vi "handleSettings.vi"(8 "error in (no error)":errorcluster, 10 "Path":path, 11 "AndorController in":refnum<class "AndorController.lvclass">) -> (0 "error out":errorcluster, 3 "AndorController out":refnum<class "AndorController.lvclass">)   [LabVIEW 2009, in "Hardware.lvlib" / "Channels.lvlib" / "AndorController.lvclass"]
uses:
  AndorController.lvclass
  CameraEventsManager/CameraEventsManger.lvclass
  CameraAcquisitor.lvclass
  CameraSettingsViewer/andorSettingsViewer.lvclass
panel:
  in  "Tab Control":T1(tab)
  in  "acquisition_mode":u16(ring)=2 caption="Acquisition Mode" items=["Single Shot"=1, "Accumulative Series"=2, "Kinetic Series"=3, "Fast Kinetic Series"=4, "Run 'till Abort"=5]
  in  "readout_mode":i16(ring)=1 caption="Readout Mode" items=["Full Vertical Binning"=0, "Single Track"=3, "Multi-Track"=1, "Random Track"=2, "Full Resolusion Image"=4]
  in  "subArea_coordinate":i32(listbox) caption="SubArea Coordinates of top left corner"
  in  "vertical_binning":dbl=1.0 caption="Vertical Binning"
  in  "horizontal_binning":dbl=1.0 caption="Horizontal Binning"
  in  "subArea_height":dbl=1024.0 caption="SubArea Height"
  in  "subArea_width":dbl=1024.0 caption="SubArea Width"
  in  "offset":dbl caption="Offset"
  in  "number_tracks":i32 caption="Number of Tracks"
  in  "track_positions":i32(listbox) caption="Track Positions"
  in  "fast_kinetic_shift_speed":dbl caption="Fast Kinetic Shift Speed"
  in  "horizontal_shift_speed":enum16{"2.5", "1", "0.05"}(ring) caption="Horizontal Shift Speed"
  in  "vertical_shift_speed":T2(ring) caption="Vertical Shift Speed"
  in  "fast_kinetic_image_number":dbl=1.0 caption="Number in fast Kinetic Series"
  in  "fast_kinetic_cycle_time":dbl caption="Fast Kinetic Cycle Time"
  in  "accumulative_cycle_time":dbl caption="Accumulative Cycle Time"
  in  "kinetic_cycle_time":dbl caption="Kinetic Cycle Time"
  in  "accumulation_image_number":dbl=1.0 caption="Number of Accumulations"
  in  "kinetic_image_number":dbl=1.0 caption="Number in Kinetic Series"
  in  "mode":enum16{"Automatic", "Hold Open", "Hold Closed"}(ring) caption="Shutter Mode"
  in  "open_time":dbl=20.0 caption="Shutter Open Time"
  in  "close_time":dbl=20.0 caption="Shutter Close Time"
  in  "exposure_time":dbl=0.02 caption="Exposure Time"
  out "start_trigger":string caption="Trigger Channel"
  in  "trigger_mode":u16(ring) caption="Trigger Mode" items=["Internal"=0, "External"=1, "Fast External"=6]
  in  "fast_trigger":bool caption="Fast Triggering"
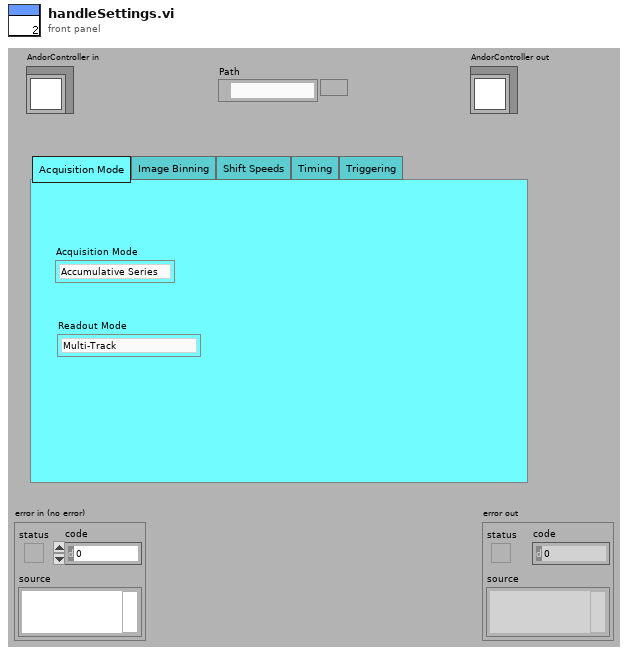
[diagram p1: front panel]
types:
  T1 = enum32{"modes", "image_binning", "shift_speeds", "timing", "triggering"}
  T2 = enum16{"0.525", "0.875", "1.575", "2.975", "5.775", "11.375", "22.575", "44.975"}
  T3 = cluster{"settingsFrontEndEvents":cluster{"loadSettingsFromPath":refnum<user-event>, "lookUpElementEvent":refnum<user-event>, "saveSettings":refnum<user-event>, "loadSettings":refnum<user-event>, "close":refnum<user-event>, "replaceElement":refnum<user-event>, "findParentNodes":refnum<user-event>, "createNode":refnum<user-event>}, "settingBackEndEvents":cluster{"defaultSettingsPathRequest":refnum<user-event>, "searchResultEvent":refnum<user-event>, "settingsSaved":refnum<user-event>, "settingsLoaded":refnum<user-event>, "foundParentNode":refnum<user-event>}}
  T4 = cluster{"loadSettingsFromPath":refnum<user-event>, "lookUpElementEvent":refnum<user-event>, "saveSettings":refnum<user-event>, "loadSettings":refnum<user-event>, "close":refnum<user-event>, "replaceElement":refnum<user-event>, "findParentNodes":refnum<user-event>, "createNode":refnum<user-event>}
  T5 = enum16{"Number", "String", "NumberArray", "StringArray", "xmlNode"}
  T6 = cluster{"[0]":dbl, "[1]":dbl, "[2]":dbl, "[3]":dbl}
  T7 = cluster{"[0]":dbl, "[1]":dbl, "[2]":dbl, "[3]":dbl, "[0]":dbl, "[1]":dbl, cluster{"[0]":i32, "[1]":i32}[], i32[]}
  T8 = cluster{"[0]":dbl, "[1]":dbl, "[2]":dbl, "[3]":dbl, "[4]":dbl, "[5]":dbl, "[6]":dbl}
  T9 = cluster{"[0]":dbl, "[1]":dbl, "[2]":dbl, "[3]":dbl, "[4]":dbl, "[5]":dbl, "[6]":dbl, dbl}
  T10 = cluster{"shutter Open Time":dbl, "Shutter Close Time":dbl, "Exposure Time":dbl, " AccumulatedCycleTime":dbl, " KineticCycleTime":dbl, "Number of Accumulations":dbl, "Number in Kinetic Series ":dbl, "Shutter Mode":dbl}
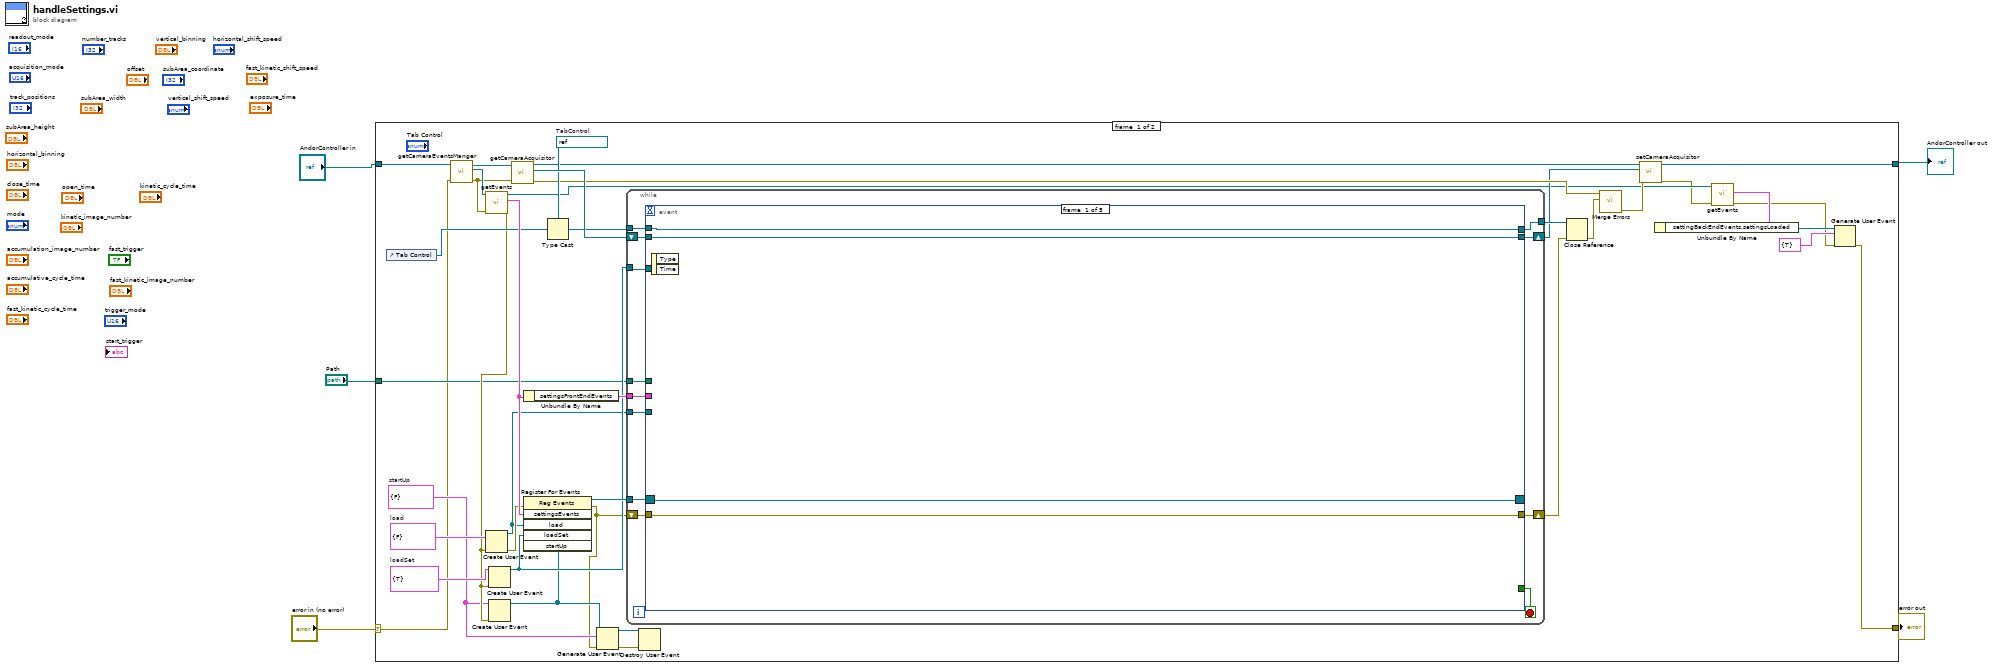
[diagram p0: block diagram]
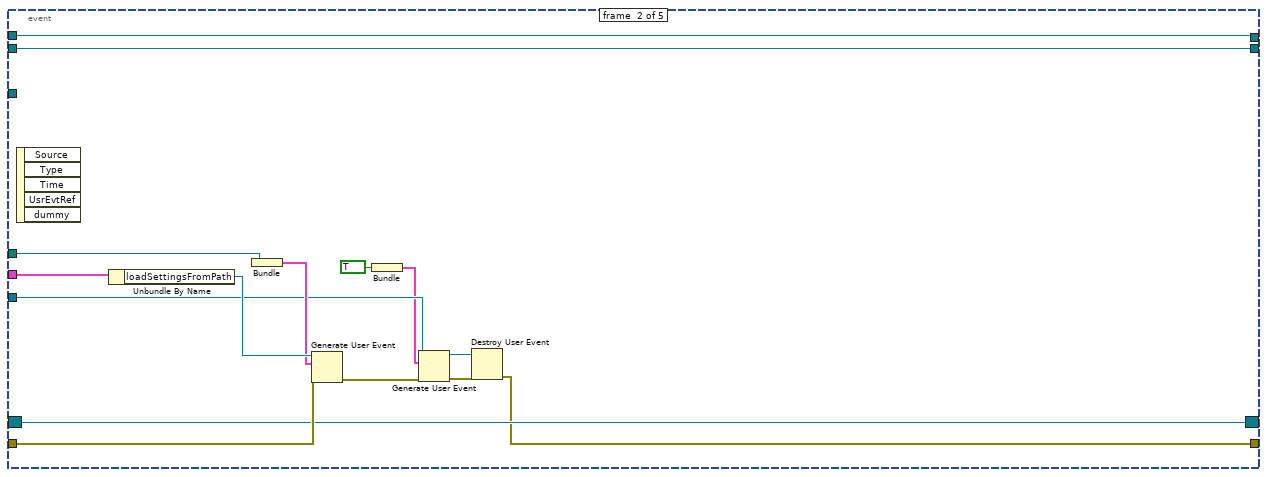
[diagram p2: hidden frame]
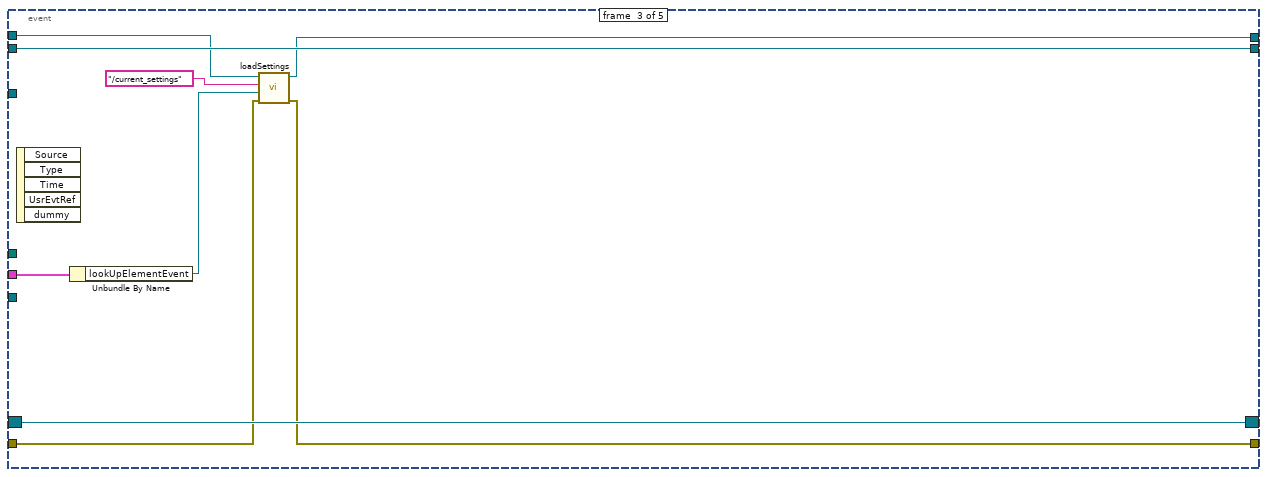
[diagram p3: hidden frame]
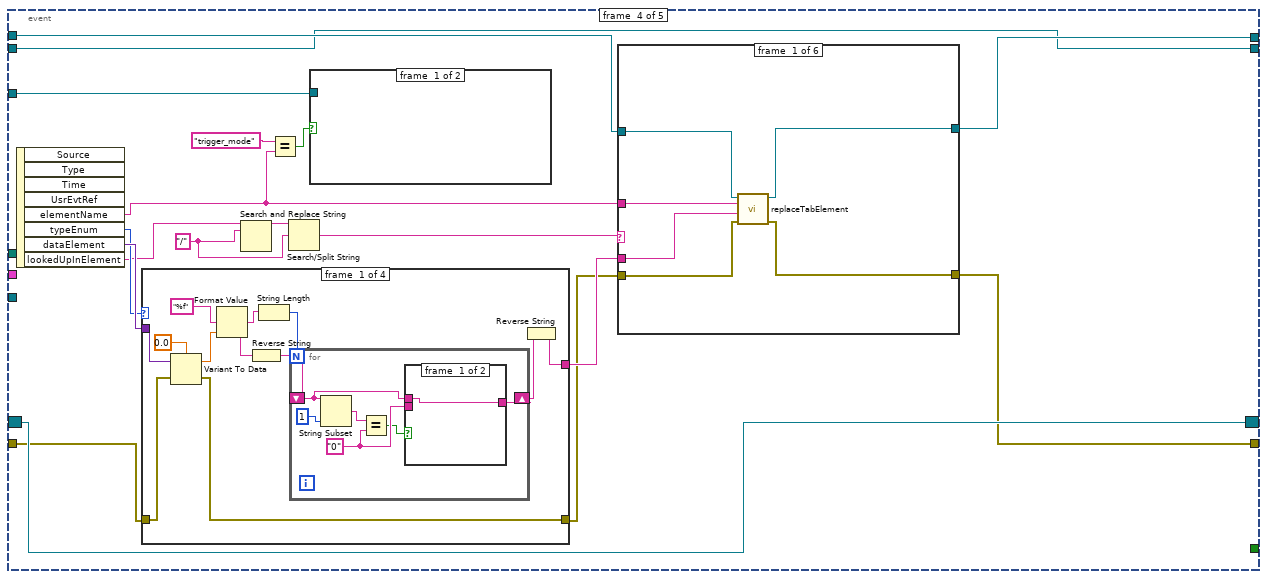
[diagram p4: hidden frame]
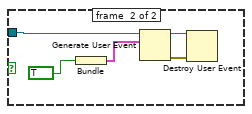
[diagram p5: hidden frame]
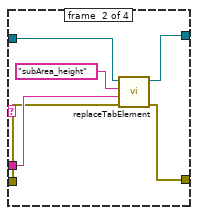
[diagram p7: hidden frame]
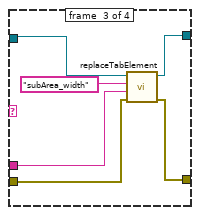
[diagram p8: hidden frame]
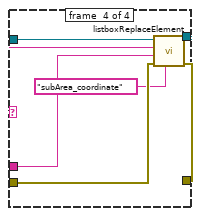
[diagram p9: hidden frame]
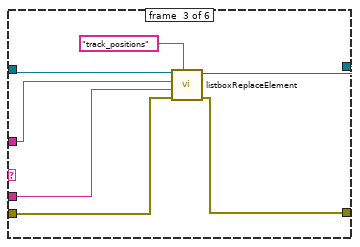
[diagram p10: hidden frame]
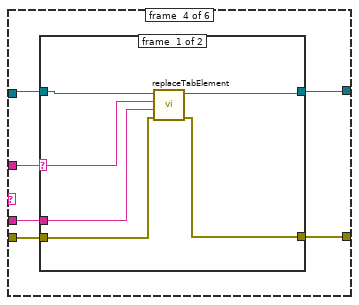
[diagram p11: hidden frame]
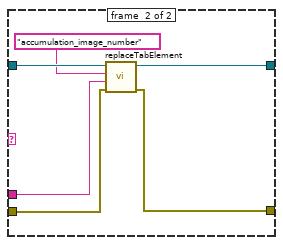
[diagram p12: hidden frame]
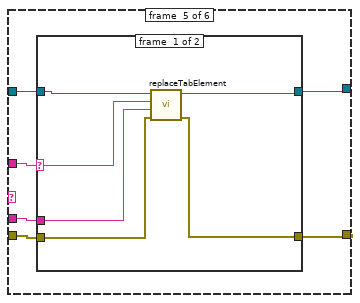
[diagram p13: hidden frame]
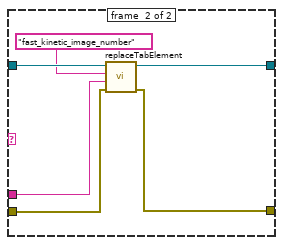
[diagram p14: hidden frame]
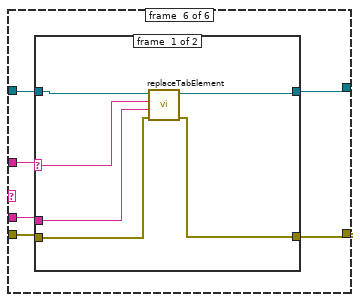
[diagram p15: hidden frame]
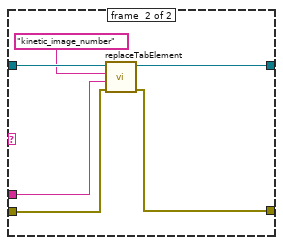
[diagram p16: hidden frame]
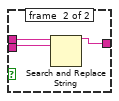
[diagram p17: hidden frame]
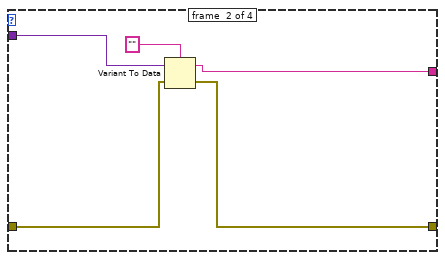
[diagram p18: hidden frame]
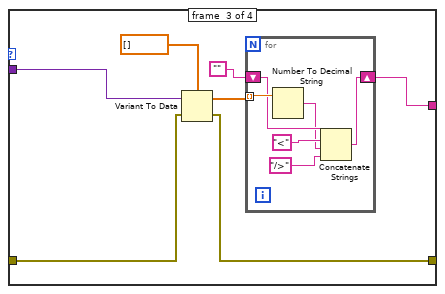
[diagram p19: hidden frame]
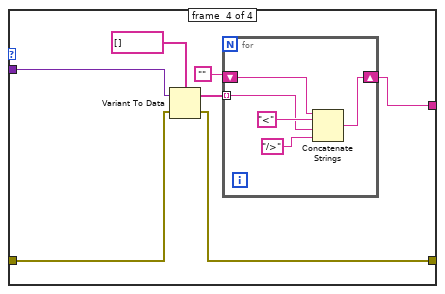
[diagram p20: hidden frame]
diagram:
  n1 = case shown="No Error" "error in (no error)" {
    selector: "error in (no error)" -> [w13 w478]
    tunnel: [w6 w478] -> w2
    tunnel: [w15 w477] -> w1
    tunnel: "AndorController in" -> [w14 w477]
    tunnel: "Path" -> [w23 _]
    frame #0 {
      w27 = cluster{"dummy":bool} {"dummy"=FALSE}  # startUp
      w33 = cluster{"dummy":bool} {"dummy"=TRUE}  # loadSet
      w36 = refnum<vi> refnum  # TabControl
      w37 = cluster{"dummy":bool} {"dummy"=FALSE}  # load
      n2 = control-ref of="Tab Control"() -> (w35:refnum<vi>)
      n3 = call-dynamic "getCameraEventsManger.vi"("error in (no error)"=w13, "CameraController.lvclass in"=w14) -> ("error out"=w39:errorcluster, "Hardware:Channels.lvlib:CameraEventsManger.lvclass"=w44:refnum<class "CameraEventsManger.lvclass">, "CameraController.lvclass out"=w40:refnum<class "AndorController.lvclass">)  [unwired: 7 in]
      n4 = call-dynamic "getEvents.vi"("error in (no error)"=w39, "CameraEventsManger in"=w44) -> ("error out"=w30:errorcluster, "settingsEvents"=w42:T3, "CameraEventsManger out"=w12:refnum<class "CameraEventsManger.lvclass">)  [unwired: 5 in, 2 out]
      n5 = Create User Event(user event datatype=w37, error in=w30) -> (user event=w29:refnum<user-event>, error out=w32:errorcluster)
      n6 = Create User Event(user event datatype=w33, error in=w30) -> (user event=w31:refnum<user-event>)  [unwired: 1 out]
      n7 = Create User Event(user event datatype=w27, error in=w30) -> (user event=w28:refnum<user-event>)  [unwired: 1 out]
      n8 = call-dynamic "getCameraAcquisitor.vi"("error in (no error)"=w39, "CameraController.lvclass in"=w40) -> ("error out"=w20:errorcluster, "CameraAcquisitor.lvclass"=w38:refnum<class "CameraAcquisitor.lvclass">, "CameraController.lvclass out"=w21:refnum<class "AndorController.lvclass">)  [unwired: 7 in]
      n9 = Unbundle By Name(w42) -> ("settingsFrontEndEvents"=w41:T4)
      n10 = register-events(error in=w32, w42, w29, w31, w28) -> (reference out=w43:refnum<event-registration>, error out=w26:errorcluster)  [unwired: 1 in]
      n11 = Type Cast(type=w36, x=w35) -> (*(type *) &x=w34:refnum<vi>)
      n12 = Generate User Event(user event=w28, event data cluster=w27, error in=w26) -> (user event out=w24:refnum<user-event>, error out=w25:errorcluster)
      n13 = while {
        tunnel: w43 -> [w56]
        shift-right: [w53] -> w18
        shift-left: w26 -> [w55]
        tunnel: w41 -> [w54]
        shift-right: [w51] -> w17
        shift-left: w38 -> [w52]
        tunnel: w29 -> [w50]
        tunnel: w34 -> [w49]
        tunnel: [w48] -> w22
        tunnel: w31 -> [w46]
        tunnel: w23 -> [w45]
        stop <- w47 stop-if-true
        n14 = event shown="[4] <loadSet>: User Event" {
          selector: w56 -> [w59 w71 w84 w102 w253]
          dyn-events: [w59 w71 w84 w102 w253] -> _
          timeout: _ -> [_ _ _ _ _]
          tunnel: w55 -> [w58 w72 w78 w100 w260]
          tunnel: w54 -> [_ w75 w80 _ _]
          tunnel: [w58 w62 w77 w93 w255] -> w53
          tunnel: w52 -> [w60 w70 w83 w94 w259]
          tunnel: [w60 w70 w83 w94 w257] -> w51
          tunnel: w50 -> [_ w69 _ _ _]
          tunnel: w49 -> [w57 w65 w82 w98 w261]
          tunnel: [w57 w65 w76 w95 w258] -> w48
          tunnel: [_ _ _ _ TRUE] -> w47
          tunnel: w46 -> [_ _ _ w89 _]
          tunnel: w45 -> [_ w64 _ _ _]
          event #0 {
            n15 = event-data() -> ()  [unwired: 1 in, 2 out]
          }
          event #1 {
            n16 = event-data() -> ()  [unwired: 1 in, 5 out]
            n17 = Unbundle By Name(w75) -> ("loadSettingsFromPath"=w74:refnum<user-event>)
            n18 = Bundle("Path"=w64) -> (w73:cluster{"Path":path})  [unwired: 1 in]
            n19 = Generate User Event(user event=w74, event data cluster=w73, error in=w72) -> (error out=w66:errorcluster)  [unwired: 1 out]
            n20 = Bundle(TRUE) -> (w67:cluster{bool})  [unwired: 1 in]
            n21 = Generate User Event(user event=w69, event data cluster=w67, error in=w66) -> (user event out=w61:refnum<user-event>, error out=w63:errorcluster)
            n22 = Destroy User Event(user event=w61, error in=w63) -> (error out=w62:errorcluster)
          }
          event #2 {
            n23 = event-data() -> ()  [unwired: 1 in, 5 out]
            n24 = Unbundle By Name(w80) -> ("lookUpElementEvent"=w79:refnum<user-event>)
            n25 = call "loadSettings.vi"("error in (no error)"=w78, "lookUpElementEvent"=w79, "whichSettings"="/current_settings", "TabCtl Refnum in"=w82) -> ("error out"=w77:errorcluster, "TabCtl Refnum out"=w76:refnum<vi>)  [unwired: 6 in]
          }
          event #3 {
            w87 = "/"
            n26 = event-data() -> ("elementName"=w91:string, "typeEnum"=w99:T5, "dataElement"=w101:variant, "lookedUpInElement"=w86:string)  [unwired: 1 in, 4 out]
            n27 = case shown="\"Number\", Default" w99 {
              tunnel: w101 -> [w209 w227 w233 w247]
              tunnel: w100 -> [w210 w226 w232 w246]
              tunnel: [w211 w225 w231 w241] -> w96
              tunnel: [w203 w223 w228 w242] -> w97
              frame #0 {
                n28 = Variant To Data(error in=w210, Variant=w209, type=0.0) -> (error out=w211:errorcluster, data=w202:dbl)
                n29 = Format Value(format string="%f", value (0)=w202) -> (output string=w205:string)  [unwired: 1 in]
                n30 = Reverse String(1:w205) -> (0:w207:string)
                n31 = String Length(string=w205) -> (length=w206:i32)
                n32 = for {
                  N: w206 -> [_]
                  shift-right: [w213] -> w204
                  shift-left: w207 -> [w216]
                  w215 = "0"
                  n33 = String Subset(string=w216, length (rest)=1) -> (substring=w217:string)  [unwired: 1 in]
                  n34 = Equal?(x=w217, y=w215) -> (x = y?=w214:bool)
                  n35 = case shown="True" w214 {
                    tunnel: w216 -> [w219 w222]
                    tunnel: w215 -> [_ w220]
                    tunnel: [w219 w221] -> w213
                    frame #0 {
                    }
                    frame #1 {
                      n36 = Search and Replace String(input string=w222, search string=w220) -> (result string=w221:string)  [unwired: 6 in, 3 out]
                    }
                  }
                }
                n37 = Reverse String(1:w204) -> (0:w203:string)
              }
              frame #1 {
                n38 = Variant To Data(error in=w226, Variant=w227, type="") -> (error out=w225:errorcluster, data=w223:string)
              }
              frame #2 {
                n39 = Variant To Data(error in=w232, Variant=w233, type=dbl[] []) -> (error out=w231:errorcluster, data=w230:dbl[])
                n40 = for {
                  tunnel: w230 -> [w240] mode=indexing
                  shift-right: [w235] -> w228
                  shift-left: "" -> [w239]
                  n41 = Number To Decimal String(number=w240) -> (decimal integer string=w237:string)  [unwired: 1 in]
                  n42 = Concatenate Strings(w239, "<", w237, "/>") -> (w235:string)
                }
              }
              frame #3 {
                n43 = Variant To Data(error in=w246, Variant=w247, type=string[] []) -> (error out=w241:errorcluster, data=w244:string[])
                n44 = for {
                  shift-right: [w248] -> w242
                  shift-left: "" -> [w249]
                  tunnel: w244 -> [w250] mode=indexing
                  n45 = Concatenate Strings(w249, "<", w250, "/>") -> (w248:string)
                }
              }
            }
            n46 = Search and Replace String(input string=w86, search string=w87) -> (result string=w88:string)  [unwired: 6 in, 3 out]
            n47 = Equal?(x="trigger_mode", y=w91) -> (x = y?=w90:bool)
            n48 = Search/Split String(string=w88, search string/char (-)=w87) -> (match + rest of string=w85:string)  [unwired: 1 in, 2 out]
            n49 = case shown="True" w90 {
              tunnel: w89 -> [_ w107]
              frame #0 {
              }
              frame #1 {
                n50 = Bundle(TRUE) -> (w105:cluster{bool})  [unwired: 1 in]
                n51 = Generate User Event(user event=w107, event data cluster=w105) -> (user event out=w103:refnum<user-event>, error out=w104:errorcluster)  [unwired: 1 in]
                n52 = Destroy User Event(user event=w103, error in=w104) -> ()  [unwired: 1 out]
              }
            }
            n53 = case shown="\"False\", Default" w85 {
              tunnel: w91 -> [w112 w114 w145 w151 w169 w187]
              tunnel: w98 -> [w113 w115 w147 w153 w171 w189]
              tunnel: w97 -> [w111 w119 w144 w152 w170 w188]
              tunnel: w96 -> [w110 w118 w142 w148 w166 w184]
              tunnel: [w109 w117 w141 w149 w167 w185] -> w93
              tunnel: [w108 w116 w146 w150 w168 w186] -> w95
              frame #0 {
                n54 = call "replaceTabElement.vi"("error in (no error)"=w110, "replaceWith"=w111, "replaceElementLabeled"=w112, "Tab ref in"=w113) -> ("error out"=w109:errorcluster, "Tab ref out"=w108:refnum<vi>)  [unwired: 6 in]
              }
              frame #1 {
                n55 = case shown="\"width\"" w114 {
                  selector: w114 -> [_ _ _ w135]
                  tunnel: w119 -> [_ w127 w129 w136]
                  tunnel: w118 -> [w120 w126 w130 w138]
                  tunnel: [w120 w125 w131 w137] -> w117
                  tunnel: [w121 w124 w132 w139] -> w116
                  tunnel: w115 -> [w121 w123 w133 w140]
                  frame #0 {
                  }
                  frame #1 {
                    n56 = call "replaceTabElement.vi"("error in (no error)"=w126, "replaceWith"=w127, "replaceElementLabeled"="subArea_height", "Tab ref in"=w123) -> ("error out"=w125:errorcluster, "Tab ref out"=w124:refnum<vi>)  [unwired: 6 in]
                  }
                  frame #2 {
                    n57 = call "replaceTabElement.vi"("error in (no error)"=w130, "replaceWith"=w129, "replaceElementLabeled"="subArea_width", "Tab ref in"=w133) -> ("error out"=w131:errorcluster, "Tab ref out"=w132:refnum<vi>)  [unwired: 6 in]
                  }
                  frame #3 {
                    n58 = call "listboxReplaceElement.vi"("inElement"="subArea_coordinate", "error in (no error)"=w138, "replaceElementWith"=w136, "elementName"=w135, "TabCtl Refnum"=w140) -> ("error out"=w137:errorcluster, "TabCtl Refnum out"=w139:refnum<vi>)  [unwired: 5 in]
                  }
                }
              }
              frame #2 {
                n59 = call "listboxReplaceElement.vi"("inElement"="track_positions", "error in (no error)"=w142, "replaceElementWith"=w144, "elementName"=w145, "TabCtl Refnum"=w147) -> ("error out"=w141:errorcluster, "TabCtl Refnum out"=w146:refnum<vi>)  [unwired: 5 in]
              }
              frame #3 {
                n60 = case shown="\"image_number\"" w151 {
                  selector: w151 -> [w158 _]
                  tunnel: w153 -> [w159 w165]
                  tunnel: w152 -> [w157 w164]
                  tunnel: [w154 w162] -> w150
                  tunnel: [w155 w161] -> w149
                  tunnel: w148 -> [w156 w160]
                  frame #0 {
                    n61 = call "replaceTabElement.vi"("error in (no error)"=w156, "replaceWith"=w157, "replaceElementLabeled"=w158, "Tab ref in"=w159) -> ("error out"=w155:errorcluster, "Tab ref out"=w154:refnum<vi>)  [unwired: 6 in]
                  }
                  frame #1 {
                    n62 = call "replaceTabElement.vi"("error in (no error)"=w160, "replaceWith"=w164, "replaceElementLabeled"="accumulation_image_number", "Tab ref in"=w165) -> ("error out"=w161:errorcluster, "Tab ref out"=w162:refnum<vi>)  [unwired: 6 in]
                  }
                }
              }
              frame #4 {
                n63 = case shown="\"image_number\"" w169 {
                  selector: w169 -> [w176 _]
                  tunnel: w171 -> [w177 w183]
                  tunnel: w170 -> [w175 w182]
                  tunnel: [w172 w180] -> w168
                  tunnel: [w173 w179] -> w167
                  tunnel: w166 -> [w174 w178]
                  frame #0 {
                    n64 = call "replaceTabElement.vi"("error in (no error)"=w174, "replaceWith"=w175, "replaceElementLabeled"=w176, "Tab ref in"=w177) -> ("error out"=w173:errorcluster, "Tab ref out"=w172:refnum<vi>)  [unwired: 6 in]
                  }
                  frame #1 {
                    n65 = call "replaceTabElement.vi"("error in (no error)"=w178, "replaceWith"=w182, "replaceElementLabeled"="fast_kinetic_image_number", "Tab ref in"=w183) -> ("error out"=w179:errorcluster, "Tab ref out"=w180:refnum<vi>)  [unwired: 6 in]
                  }
                }
              }
              frame #5 {
                n66 = case shown="\"False\", Default" w187 {
                  selector: w187 -> [w194 _]
                  tunnel: w189 -> [w195 w201]
                  tunnel: w188 -> [w193 w200]
                  tunnel: [w190 w198] -> w186
                  tunnel: [w191 w197] -> w185
                  tunnel: w184 -> [w192 w196]
                  frame #0 {
                    n67 = call "replaceTabElement.vi"("error in (no error)"=w192, "replaceWith"=w193, "replaceElementLabeled"=w194, "Tab ref in"=w195) -> ("error out"=w191:errorcluster, "Tab ref out"=w190:refnum<vi>)  [unwired: 6 in]
                  }
                  frame #1 {
                    n68 = call "replaceTabElement.vi"("error in (no error)"=w196, "replaceWith"=w200, "replaceElementLabeled"="kinetic_image_number", "Tab ref in"=w201) -> ("error out"=w197:errorcluster, "Tab ref out"=w198:refnum<vi>)  [unwired: 6 in]
                  }
                }
              }
            }
          }
          event #4 {
            n69 = event-data() -> ()  [unwired: 1 in, 5 out]
            n70 = for {
              N: 3 -> [_]
              shift-right: [w263] -> w258
              shift-left: w261 -> [w267]
              shift-right: [w262] -> w255
              shift-left: w260 -> [w266]
              shift-right: [w264] -> w257
              shift-left: w259 -> [w265]
              i -> [w268]
              n71 = case shown="1" w268 {
                tunnel: w267 -> [w269 w346 w398 w473]
                tunnel: w266 -> [w270 w345 w397 w443]
                tunnel: w265 -> [w271 w331 w370 w457]
                tunnel: [w271 w283 w369 w429] -> w264
                tunnel: [w269 w282 w375 w440] -> w263
                tunnel: [w270 w280 w371 w428] -> w262
                frame #0 {
                }
                frame #1 {
                  w297 = refnum<vi> refnum  # MulticolumnListbox
                  w302 = refnum<vi> refnum  # MulticolumnListbox
                  n72 = call "findTabElement.vi"("error in (no error)"=w345, "replaceElementLabeled"="acquisition_mode", "Tab ref in"=w346) -> ("error out"=w341:errorcluster, "Tab Control"=w337:refnum<vi>, "Tab ref out"=w343:refnum<vi>)  [unwired: 5 in, 1 out]
                  n73 = call "findTabElement.vi"("error in (no error)"=w341, "replaceElementLabeled"="readout_mode", "Tab ref in"=w343) -> ("error out"=w339:errorcluster, "Tab Control"=w336:refnum<vi>, "Tab ref out"=w340:refnum<vi>)  [unwired: 5 in, 1 out]
                  n74 = Build Array(w337, w336) -> (w332:refnum<vi>[])
                  n75 = call "findTabElement.vi"("error in (no error)"=w339, "replaceElementLabeled"="vertical_binning", "Tab ref in"=w340) -> ("error out"=w334:errorcluster, "Tab Control"=w312:refnum<vi>, "Tab ref out"=w335:refnum<vi>)  [unwired: 5 in, 1 out]
                  n76 = for {
                    tunnel: w332 -> [w357] mode=indexing
                    tunnel: [w356] -> w278 mode=indexing
                    n77 = call "getNumber.vi"("Tab Control"=w357) -> ("Number"=w356:dbl)  [unwired: 9 in, 1 out]
                  }
                  n78 = call "findTabElement.vi"("error in (no error)"=w334, "replaceElementLabeled"="horizontal_binning", "Tab ref in"=w335) -> ("error out"=w330:errorcluster, "Tab Control"=w311:refnum<vi>, "Tab ref out"=w328:refnum<vi>)  [unwired: 5 in, 1 out]
                  n79 = call "findTabElement.vi"("error in (no error)"=w330, "replaceElementLabeled"="subArea_height", "Tab ref in"=w328) -> ("error out"=w326:errorcluster, "Tab Control"=w310:refnum<vi>, "Tab ref out"=w327:refnum<vi>)  [unwired: 5 in, 1 out]
                  n80 = Index Array(array=w278) -> (element=w277:dbl)  [unwired: 1 in]
                  n81 = Index Array(array=w278, index=1) -> (element=w276:dbl)
                  n82 = call "findTabElement.vi"("error in (no error)"=w326, "replaceElementLabeled"="subArea_width", "Tab ref in"=w327) -> ("error out"=w324:errorcluster, "Tab Control"=w309:refnum<vi>, "Tab ref out"=w322:refnum<vi>)  [unwired: 5 in, 1 out]
                  n83 = Build Array(w312, w311, w310, w309) -> (w307:refnum<vi>[])
                  n84 = Bundle("Number"=w277, "Number"=w276, 0.0) -> (w274:cluster{"Number":dbl, "Number":dbl, dbl})  [unwired: 1 in]
                  n85 = call "findTabElement.vi"("error in (no error)"=w324, "replaceElementLabeled"="subArea_coordinate", "Tab ref in"=w322) -> ("error out"=w320:errorcluster, "Tab Control"=w303:refnum<vi>, "Tab ref out"=w321:refnum<vi>)  [unwired: 5 in, 1 out]
                  n86 = Type Cast(type=w302, x=w303) -> (*(type *) &x=w304:refnum<vi>)
                  n87 = for {
                    tunnel: w307 -> [w355] mode=indexing
                    tunnel: [w354] -> w308 mode=indexing
                    n88 = call "getNumber.vi"("Tab Control"=w355) -> ("Number"=w354:dbl)  [unwired: 9 in, 1 out]
                  }
                  n89 = call "findTabElement.vi"("error in (no error)"=w320, "replaceElementLabeled"="offset", "Tab ref in"=w321) -> ("error out"=w316:errorcluster, "Tab Control"=w273:refnum<vi>, "Tab ref out"=w317:refnum<vi>)  [unwired: 5 in, 1 out]
                  n90 = property class="MCListbox"(reference=w304) -> ("ItemNames"=w301:string[][])  [unwired: 1 in, 2 out]
                  n91 = call "findTabElement.vi"("error in (no error)"=w316, "replaceElementLabeled"="number_tracks", "Tab ref in"=w317) -> ("error out"=w314:errorcluster, "Tab Control"=w272:refnum<vi>, "Tab ref out"=w315:refnum<vi>)  [unwired: 5 in, 1 out]
                  n92 = Array To Cluster(array=w308) -> (cluster=w294:T6)
                  n93 = Build Array(w273, w272) -> (w305:refnum<vi>[])
                  n94 = call "findTabElement.vi"("error in (no error)"=w314, "replaceElementLabeled"="track_positions", "Tab ref in"=w315) -> ("error out"=w281:errorcluster, "Tab Control"=w295:refnum<vi>, "Tab ref out"=w282:refnum<vi>)  [unwired: 5 in, 1 out]
                  n95 = Type Cast(type=w297, x=w295) -> (*(type *) &x=w298:refnum<vi>)
                  n96 = Decimal String To Number(string=w301) -> (number=w300:i32[][])  [unwired: 2 in, 1 out]
                  n97 = property class="MCListbox"(reference=w298) -> ("ItemNames"=w296:string[][])  [unwired: 1 in, 2 out]
                  n98 = for {
                    tunnel: w305 -> [w353] mode=indexing
                    tunnel: [w352] -> w306 mode=indexing
                    n99 = call "getNumber.vi"("Tab Control"=w353) -> ("Number"=w352:dbl)  [unwired: 9 in, 1 out]
                  }
                  n100 = Reshape Array(w300, 2) -> (w285:i32[])
                  n101 = Array To Cluster(array=w306) -> (cluster=w293:cluster{"[0]":dbl, "[1]":dbl})
                  n102 = for {
                    tunnel: w296 -> [w351] mode=indexing
                    tunnel: [w347] -> w286 mode=indexing
                    n103 = Decimal String To Number(string=w351) -> (number=w350:i32[])  [unwired: 2 in, 1 out]
                    n104 = Reshape Array(w350, 2) -> (w348:i32[])
                    n105 = Array To Cluster(array=w348) -> (cluster=w347:cluster{"[0]":i32, "[1]":i32})
                  }
                  n106 = Unbundle(w293) -> ("[0]"=w288:dbl, "[1]"=w287:dbl)
                  n107 = Unbundle(w294) -> ("[0]"=w292:dbl, "[1]"=w291:dbl, "[2]"=w290:dbl, "[3]"=w289:dbl)
                  n108 = Bundle("[0]"=w292, "[1]"=w291, "[2]"=w290, "[3]"=w289, "[0]"=w288, "[1]"=w287, w286, w285) -> (w284:T7)  [unwired: 1 in]
                  n109 = call "configureImageAcquisition.vi"("error in (no error)"=w281, "Image Binning"=w284, "Mode"=w274, "CameraAcquisitor in"=w331) -> ("error out"=w280:errorcluster, "CameraAcquisitor out"=w283:refnum<class "CameraAcquisitor.lvclass">)  [unwired: 6 in]
                }
                frame #2 {
                  w390 = refnum<vi> refnum  # Enum
                  n110 = Build Array("open_time", "close_time", "exposure_time", "accumulative_cycle_time", "kinetic_cycle_time", "accumulation_image_number", "kinetic_image_number") -> (w399:string[])
                  n111 = for {
                    tunnel: w399 -> [w424] mode=indexing
                    shift-right: [w418] -> w395
                    shift-left: w398 -> [w425]
                    shift-right: [w419] -> w393
                    shift-left: w397 -> [w423]
                    tunnel: [w420] -> w396 mode=indexing
                    n112 = call "findTabElement.vi"("error in (no error)"=w423, "replaceElementLabeled"=w424, "Tab ref in"=w425) -> ("error out"=w421:errorcluster, "Tab Control"=w422:refnum<vi>, "Tab ref out"=w418:refnum<vi>)  [unwired: 5 in, 1 out]
                    n113 = call "getNumber.vi"("error in (no error)"=w421, "Tab Control"=w422) -> ("error out"=w419:errorcluster, "Number"=w420:dbl)  [unwired: 8 in]
                  }
                  n114 = Build Array("vertical_shift_speed", "horizontal_shift_speed") -> (w376:string[])
                  n115 = Array To Cluster(array=w396) -> (cluster=w388:T8)
                  n116 = call "findTabElement.vi"("error in (no error)"=w393, "replaceElementLabeled"="mode", "Tab ref in"=w395) -> ("error out"=w366:errorcluster, "Tab Control"=w391:refnum<vi>, "Tab ref out"=w367:refnum<vi>)  [unwired: 5 in, 1 out]
                  n117 = Type Cast(type=w390, x=w391) -> (*(type *) &x=w392:refnum<vi>)
                  n118 = for {
                    tunnel: w376 -> [w416] mode=indexing
                    shift-right: [w412] -> w375
                    shift-left: w367 -> [w417]
                    shift-right: [w407] -> w373
                    shift-left: w366 -> [w415]
                    tunnel: [w408] -> w363 mode=indexing
                    w414 = refnum<vi> refnum  # Enum
                    n119 = call "findTabElement.vi"("error in (no error)"=w415, "replaceElementLabeled"=w416, "Tab ref in"=w417) -> ("error out"=w410:errorcluster, "Tab Control"=w413:refnum<vi>, "Tab ref out"=w412:refnum<vi>)  [unwired: 5 in, 1 out]
                    n120 = Type Cast(type=w414, x=w413) -> (*(type *) &x=w411:refnum<vi>)
                    n121 = property class="Enum"(reference=w411, error in=w410) -> (error out=w407:errorcluster, "RingText.Text"=w409:string)  [unwired: 1 out]
                    n122 = Fract/Exp String To Number(string=w409) -> (number=w408:dbl)  [unwired: 3 in, 1 out]
                  }
                  n123 = call "findTabElement.vi"("error in (no error)"=w366, "replaceElementLabeled"="fast_kinetic_shift_speed", "Tab ref in"=w367) -> ("error out"=w364:errorcluster, "Tab Control"=w365:refnum<vi>)  [unwired: 5 in, 2 out]
                  n124 = property class="Enum"(reference=w392, error in=w366) -> (error out=w374:errorcluster, "DigDisp.Text"=w389:string)  [unwired: 1 out]
                  n125 = Unbundle(w388) -> ("[0]"=w387:dbl, "[1]"=w386:dbl, "[2]"=w385:dbl, "[3]"=w384:dbl, "[4]"=w382:dbl, "[5]"=w383:dbl, "[6]"=w381:dbl)
                  n126 = call "getNumber.vi"("error in (no error)"=w364, "Tab Control"=w365) -> ("Number"=w362:dbl)  [unwired: 8 in, 1 out]
                  n127 = Fract/Exp String To Number(string=w389) -> (number=w380:dbl)  [unwired: 3 in, 1 out]
                  n128 = Bundle("[0]"=w387, "[1]"=w386, "[2]"=w385, "[3]"=w384, "[4]"=w382, "[5]"=w383, "[6]"=w381, w380) -> (w379:T9)  [unwired: 1 in]
                  n129 = Array To Cluster(array=w363) -> (cluster=w360:cluster{"[0]":dbl, "[1]":dbl})
                  n130 = call <vilib>:"Merge Errors.vi"("error in 2 (no error)"=w373, "error in 1 (no error)"=w374) -> ("error out"=w372:errorcluster)  [unwired: 5 in]
                  n131 = Unbundle(w360) -> ("[0]"=w359:dbl, "[1]"=w358:dbl)
                  n132 = Bundle("[0]"=w359, "[1]"=w358, "Number"=w362) -> (w361:cluster{"[0]":dbl, "[1]":dbl, "Number":dbl})  [unwired: 1 in]
                  n133 = call "configureImageTiming.vi"("error in (no error)"=w372, "Shift Speed"=w361, "Timing"=w379, "CameraAcquisitor in"=w370) -> ("error out"=w371:errorcluster, "CameraAcquisitor out"=w369:refnum<class "CameraAcquisitor.lvclass">)  [unwired: 6 in]
                }
                frame #3 {
                  w434 = refnum<vi> refnum  # String
                  w464 = refnum<vi> refnum  # Boolean
                  w472 = refnum<vi> refnum  # Ring
                  n134 = call-dynamic "getTiming.vi"("error in (no error)"=w443, "CameraAcquisitor.lvclass in"=w457) -> ("error out"=w442:errorcluster, "Timing"=w455:T10, "CameraAcquisitor.lvclass out"=w448:refnum<class "CameraAcquisitor.lvclass">)  [unwired: 7 in]
                  n135 = call "findTabElement.vi"("error in (no error)"=w442, "replaceElementLabeled"="trigger_mode", "Tab ref in"=w473) -> ("error out"=w475:errorcluster, "Tab Control"=w476:refnum<vi>, "Tab ref out"=w467:refnum<vi>)  [unwired: 5 in, 1 out]
                  n136 = Unbundle By Name(w455) -> ("Number of Accumulations"=w452:dbl, "Number in Kinetic Series"=w450:dbl)
                  n137 = Type Cast(type=w472, x=w476) -> (*(type *) &x=w471:refnum<vi>)
                  n138 = property class="Ring"(reference=w471, error in=w475) -> (error out=w465:errorcluster, "RingText.Text"=w469:string, "Strings []"=w470:string[])  [unwired: 1 out]
                  n139 = Equal To 0?(x=w452) -> (x = 0?=w454:bool)
                  n140 = Search 1D Array(1D array=w470, element=w469) -> (index of element=w468:i32)  [unwired: 1 in]
                  n141 = Select(t=1, s=w454, f=w452) -> (s? t:f=w451:dbl)
                  n142 = Multiply(x=w451, y=w450) -> (x*y=w446:dbl)
                  n143 = Equal To 0?(x=w446) -> (x = 0?=w449:bool)
                  n144 = call "findTabElement.vi"("error in (no error)"=w465, "replaceElementLabeled"="fast_trigger", "Tab ref in"=w467) -> ("error out"=w456:errorcluster, "Tab Control"=w463:refnum<vi>, "Tab ref out"=w441:refnum<vi>)  [unwired: 5 in, 1 out]
                  n145 = Select(t=1, s=w449, f=w446) -> (s? t:f=w445:dbl)
                  n146 = Type Cast(type=w464, x=w463) -> (*(type *) &x=w462:refnum<vi>)
                  n147 = property class="Bool"(reference=w462, error in=w456) -> (error out=w459:errorcluster, "Value"=w461:variant)  [unwired: 1 out]
                  n148 = Variant To Data(error in=w459, Variant=w461, type=TRUE) -> (error out=w438:errorcluster, data=w458:bool)
                  n149 = Bundle("index of element"=w468, w458) -> (w444:cluster{"index of element":i32, bool})  [unwired: 1 in]
                  n150 = call "findTabElement.vi"("error in (no error)"=w438, "replaceElementLabeled"="start_trigger", "Tab ref in"=w441) -> ("error out"=w435:errorcluster, "Tab Control"=w437:refnum<vi>, "Tab ref out"=w440:refnum<vi>)  [unwired: 5 in, 1 out]
                  n151 = Type Cast(type=w434, x=w437) -> (*(type *) &x=w436:refnum<vi>)
                  n152 = property class="Str"(reference=w436, error in=w435) -> (reference out=w433:refnum<vi>, error out=w432:errorcluster, "Value"=w426:string)
                  n153 = Close Reference(reference=w433, error in (no error)=w432) -> (error out=w431:errorcluster)
                  n154 = call "configureImageTriggering.vi"("error in (no error)"=w431, "Number of Images"=w445, "Triggering"=w444, "CameraAcquisitor in"=w448) -> ("error out"=w427:errorcluster, "CameraAcquisitor out"=w430:refnum<class "CameraAcquisitor.lvclass">)  [unwired: 6 in]
                  n155 = call-dynamic "setStart_trigger.vi"("error in (no error)"=w427, "start_trigger"=w426, "CameraAcquisitor.lvclass in"=w430) -> ("error out"=w428:errorcluster, "CameraAcquisitor.lvclass out"=w429:refnum<class "CameraAcquisitor.lvclass">)  [unwired: 7 in]
                }
              }
            }
          }
        }
      }
      n156 = Destroy User Event(user event=w24, error in=w25) -> ()  [unwired: 1 out]
      n157 = Close Reference(reference=w22, error in (no error)=w18) -> (error out=w19:errorcluster)
      n158 = call <vilib>:"Merge Errors.vi"("error in 2 (no error)"=w19, "error in 1 (no error)"=w20) -> ("error out"=w16:errorcluster)  [unwired: 5 in]
      n159 = call-dynamic "setCameraAcquisitor.vi"("error in (no error)"=w16, "Hardware:Channels.lvlib:CameraAcquisitor.lvclass"=w17, "CameraController.lvclass in"=w21) -> ("error out"=w11:errorcluster, "CameraController.lvclass out"=w15:refnum<class "AndorController.lvclass">)  [unwired: 7 in]
      n160 = call-dynamic "getEvents.vi"("error in (no error)"=w11, "CameraEventsManger in"=w12) -> ("error out"=w7:errorcluster, "settingsEvents"=w10:T3)  [unwired: 5 in, 3 out]
      n161 = Unbundle By Name(w10) -> ("settingBackEndEvents.settingsLoaded"=w9:refnum<user-event>)
      n162 = Generate User Event(user event=w9, event data cluster=cluster{"Dummy":bool} {"Dummy"=TRUE} ("event data"), error in=w7) -> (error out=w6:errorcluster)  [unwired: 1 out]
    }
    frame #1 {
    }
  }
  "error out" <- w2
  "AndorController out" <- w1
